vi "SVI_CO_Parser.vi"(0 "read buffer":string, 1 "Time Step (ms)":i32, 3 "In":T1) -> (5 "Current Values":T3, 8 "Out":T2)   [LabVIEW 2014]
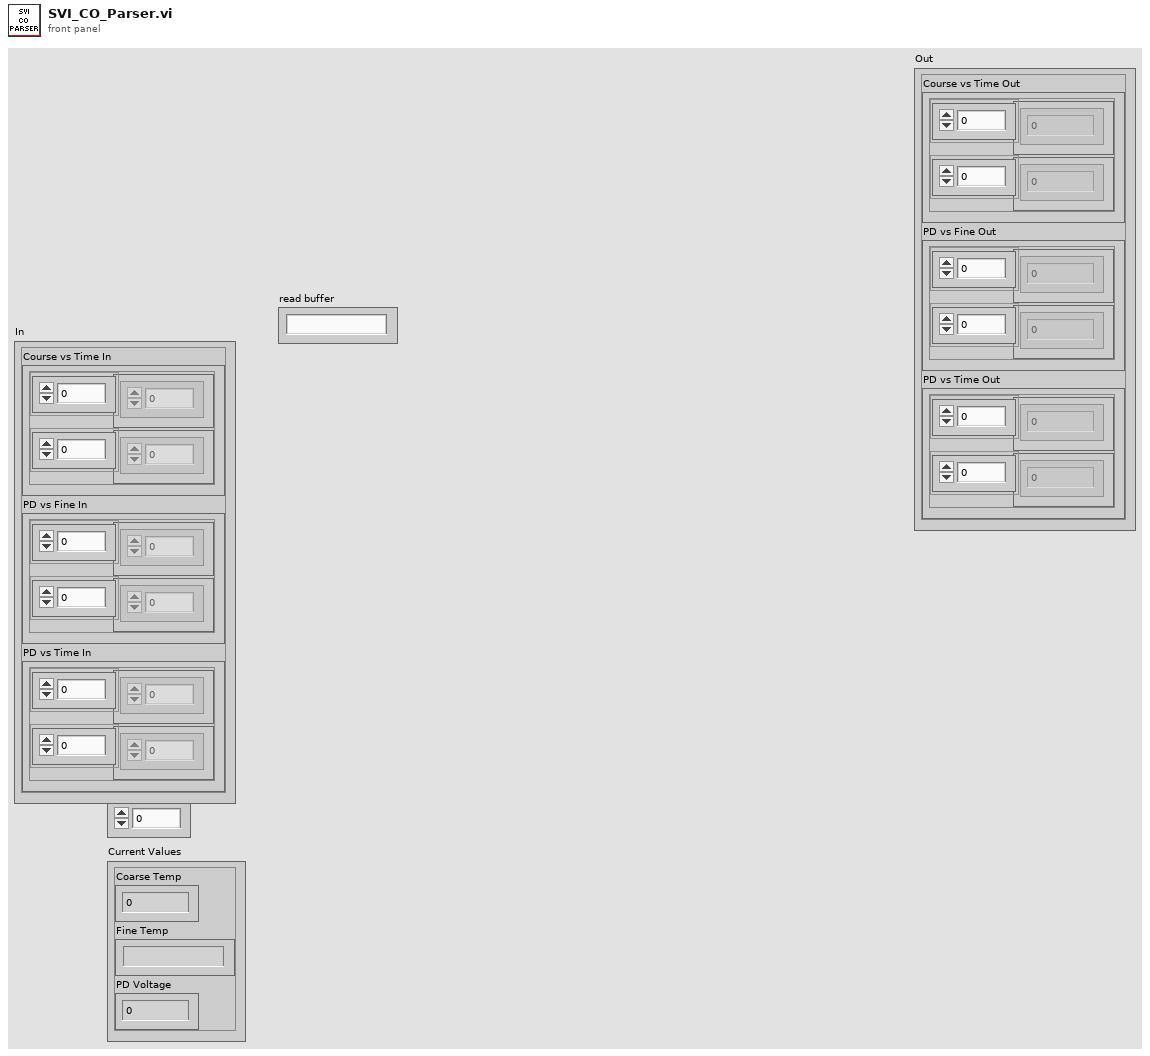
[diagram p1: front panel]
types:
  T1 = cluster{"Course vs Time In":cluster{"Array":dbl[], "Array":dbl[]}, "PD vs Fine In":cluster{"Array":dbl[], "Array":dbl[]}, "PD vs Time In":cluster{"Array":dbl[], "Array":dbl[]}}
  T2 = cluster{"Course vs Time Out":cluster{"Array":dbl[], "Array":dbl[]}, "PD vs Fine Out":cluster{"Array":dbl[], "Array":dbl[]}, "PD vs Time Out":cluster{"Array":dbl[], "Array":dbl[]}}
  T3 = cluster{"Coarse Temp":dbl, "Fine Temp":string, "PD Voltage":dbl}
  T4 = cluster{"Cluster":cluster{"Array":dbl[], "Array":dbl[]}, "PD vs Fine Temp In":cluster{"Array":dbl[], "Array":dbl[]}, "Cluster":cluster{"Array":dbl[], "Array":dbl[]}}
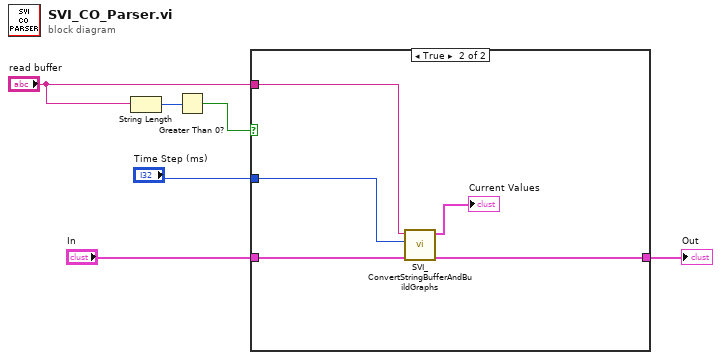
[diagram p0: block diagram]
diagram:
  n1 = String Length(string="read buffer") -> (length=w6:i32)
  n2 = Greater Than 0?(x=w6) -> (x > 0?=w5:bool)
  n3 = case shown="True" w5 {
    tunnel: "read buffer" -> [_ w10]
    tunnel: "Time Step (ms)" -> [_ w11]
    tunnel: "In" -> [w7 w9]
    tunnel: [w7 w8] -> w1
    frame False {
    }
    frame True {
      n4 = call "SVI_ConvertStringBufferAndBuildGraphs.vi"("Graphs In"=w9, "Time Step (ms)"=w11, "buffer"=w10) -> ("Graphs Out"=w8:T4, "Current Values"=→"Current Values":T3)  [unwired: 7 in]
    }
  }
  "Out" <- w1
